vi "set joystick settings.vi"(8 "error in (no error)":errorcluster, 10 "joystick_settings":T1, 11 "id":i32) -> (0 "error out":errorcluster, 3 "function return":i32)   [LabVIEW 2012, in "libximc.lvlib"]
doc: "result_t XIMC_API set_joystick_settings (device_t id, const joystick_settings_t* joystick_settings);"
uses:
  libximc.lvlib
  libximc.dll
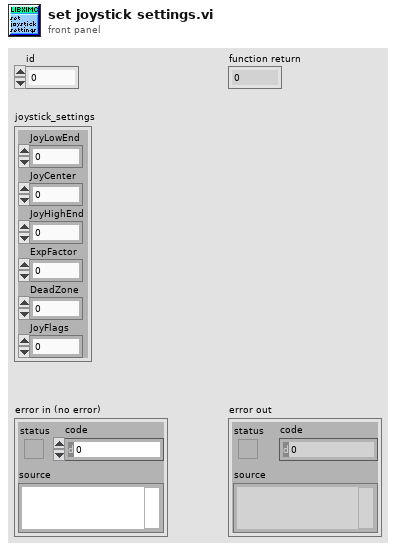
[diagram p1: front panel]
types:
  T1 = cluster{"JoyLowEnd":u32, "JoyCenter":u32, "JoyHighEnd":u32, "ExpFactor":u32, "DeadZone":u32, "JoyFlags":u32}
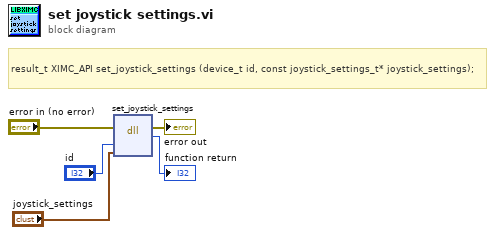
[diagram p0: block diagram]
diagram:
  # "result_t XIMC_API set_joystick_settings (device_t id, const joystick_settings_t* joystick_settings);"
  n1 = dll-call lib="E:/labview-2.12.1-Labview_12.0/ximcLVx32/libximc.*" fn="set_joystick_settings"(error in="error in (no error)", "id"="id", "joystick_settings"="joystick_settings") -> (error out=→"error out":errorcluster, →"function return":i32)  [unwired: 4 in, 1 out]
